vi "wczytajYZ.vi"(7 "Liczba bajtów":u8, 8 "error in (no error)":errorcluster, 9 "I2C Adres":u8, 10 "I2C Kana³":u8, 11 "LINX Resource in":T1) -> (0 "error out":errorcluster, 1 "Oœ Z":dbl[](array[numeric]), 2 "Oœ Y":dbl[](array[numeric]), 3 "LINX Resource out":T1)   [LabVIEW 2014]
uses:
  <vilib>/MakerHub/LINX/Private/Type Defs/LINX Ref.ctl
  <vilib>/MakerHub/LINX/Private/Type Defs/Platform.ctl
  <vilib>/MakerHub/LINX/Private/Type Defs/Interface.ctl
  <vilib>/MakerHub/LINX/Private/Device/Type Defs/LINX Device Config.ctl
  <vilib>/MakerHub/LINX/Private/Device/Type Defs/TCP Config.ctl
  <vilib>/MakerHub/LINX/Private/Device/Type Defs/Channels.ctl
  <vilib>/MakerHub/LINX/Private/Type Defs/Peripherals/I2C/EOF.ctl
  <vilib>/MakerHub/LINX/Private/Local IO/LinxI2cWrite.vi
  <vilib>/MakerHub/LINX/Public/Utilities/Check Channel.vi
  <vilib>/MakerHub/LINX/Private/Local IO/Handle Errors.vi
  <vilib>/MakerHub/LINX/Private/Utilties/Generate Error.vi
  <vilib>/MakerHub/LINX/LMH-LINX.lvlib
  <vilib>/MakerHub/LINX/Private/Device/Device.lvlib
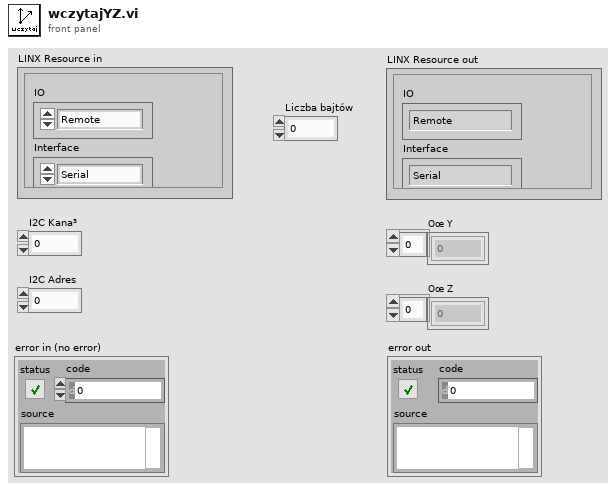
[diagram p1: front panel]
types:
  T1 = typedef "LMH-LINX.lvlib/LINX Ref.ctl" = cluster{"IO":T2, "Interface":T3, "LINX Device Config":T4}
  T2 = typedef "LMH-LINX.lvlib/Platform.ctl" = enum16{"Remote", "Local"}
  T3 = typedef "LMH-LINX.lvlib/Interface.ctl" = enum16{"Serial", "TCP"}
  T4 = typedef "LMH-LINX.lvlib/Device.lvlib/LINX Device Config.ctl" = cluster{"Interface":T3, "COM Port":refnum<visa-resource-name>, "TCP Configuration":T5, "Device Family":u8, "Device ID":u8, "Device Name":string, "TCP Ref":refnum<k5>, "Channels":T6}
  T5 = typedef "LMH-LINX.lvlib/Device.lvlib/TCP Config.ctl" = cluster{"IP Address":string, "Port":u16}
  T6 = typedef "LMH-LINX.lvlib/Channels.ctl" = cluster{"DI":u8[], "DO":u8[], "AI":u8[], "AO":u8[], "PWM":u8[], "QE":u8[], "UART":u8[], "I2C 2":u8[], "SPI":u8[], "CAN":u8[], "Servo":u8[], "AI Ref (V)":dbl, "AI Resolution (Bits)":u8, "AO Ref (V)":dbl, "AO Resolution (Bits)":u8}
  T7 = typedef "LMH-LINX.lvlib/EOF.ctl" = enum8{"Stop", "Restart", "Restart No Stop", "No Stop"}
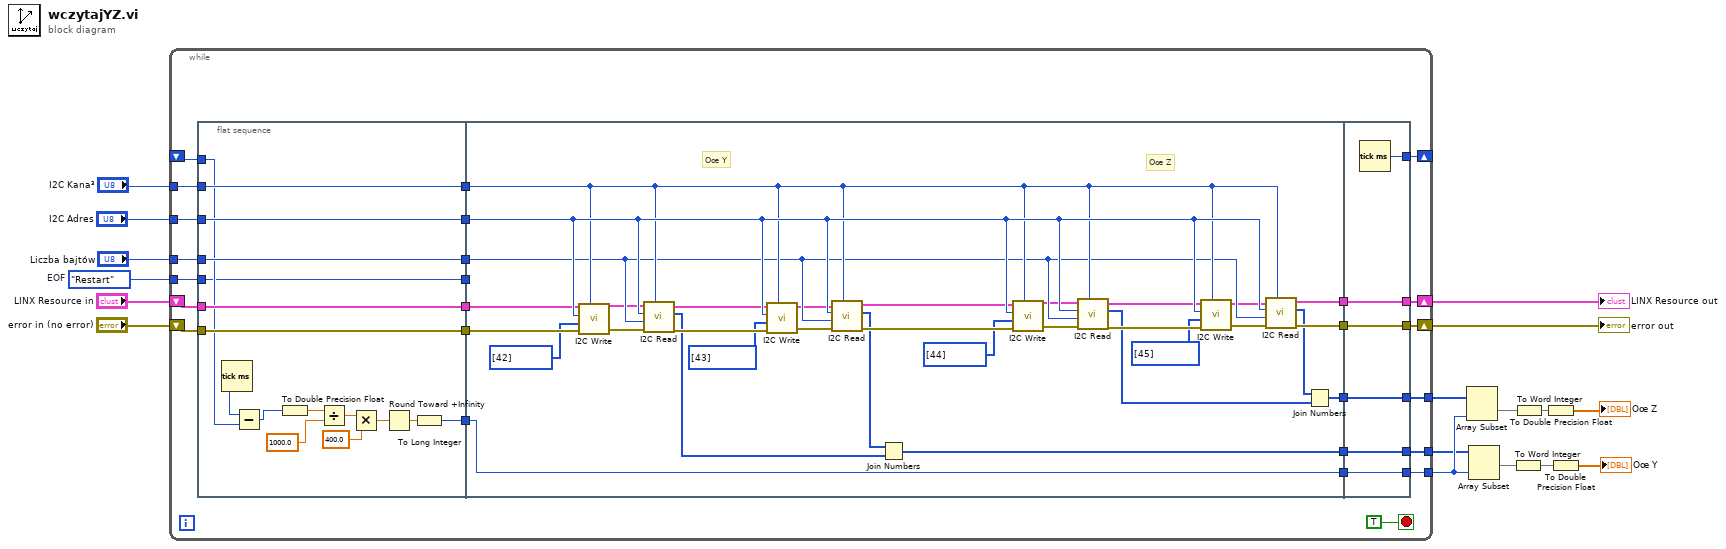
[diagram p0: block diagram]
diagram:
  w1 = EOF."Restart"  # EOF
  n1 = while {
    tunnel: "I2C Adres" -> [w43]
    tunnel: "I2C Kana³" -> [w42]
    tunnel: "Liczba bajtów" -> [w41]
    tunnel: [w38] -> w2
    tunnel: [w35] -> w10
    shift-right: [w36] -> w9
    shift-left: "LINX Resource in" -> [w40]
    shift-right: [w37] -> w8
    shift-left: "error in (no error)" -> [w39]
    shift-right: [w30] -> _
    shift-left: _ -> [w23]
    tunnel: [w20] -> w17
    tunnel: w1 -> [w18]
    stop <- TRUE stop-if-true
    n2 = flat-sequence {
      tunnel: w39 -> [w55]
      tunnel: w40 -> [w56]
      tunnel: w41 -> [w57]
      tunnel: w42 -> [w58]
      tunnel: w43 -> [w59]
      tunnel: [w59] -> w28
      tunnel: [w58] -> w27
      tunnel: [w57] -> w26
      tunnel: [w56] -> w25
      tunnel: [w55] -> w24
      tunnel: w23 -> [w50]
      tunnel: [w49] -> w22
      tunnel: [w44] -> w19
      tunnel: w18 -> [w44]
      tunnel: [w86] -> w34
      tunnel: [w85] -> w33
      tunnel: [w84] -> w32
      tunnel: [w60] -> w31
      tunnel: w28 -> [w91]
      tunnel: w27 -> [w90]
      tunnel: w26 -> [w89]
      tunnel: w25 -> [w88]
      tunnel: w24 -> [w87]
      tunnel: w22 -> [w63]
      tunnel: [w63] -> w21
      tunnel: w19 -> [_]
      tunnel: [w94] -> w35
      tunnel: [w95] -> w36
      tunnel: [w96] -> w37
      tunnel: [w97] -> w38
      tunnel: w34 -> [w97]
      tunnel: w33 -> [w96]
      tunnel: w32 -> [w95]
      tunnel: w31 -> [w94]
      tunnel: [w93] -> w30
      tunnel: [w92] -> w20
      tunnel: w21 -> [w92]
      frame #0 {
        n3 = Tick Count (ms)() -> (millisecond timer value=w51:u32)
        n4 = Subtract(x=w51, y=w50) -> (x-y=w47:u32)
        n5 = To Double Precision Float(number=w47) -> (double precision float=w46:dbl)
        n6 = Divide(x=w46, y=1000.0 ("x")) -> (x/y=w48:dbl)
        n7 = Multiply(x=w48, y=400.0) -> (x*y=w53:dbl)
        n8 = Round Toward +Infinity(x=w53) -> (ceil(x): smallest int >= x=w54:dbl)
        n9 = To Long Integer(number=w54) -> (32bit integer=w49:i32)
      }
      frame #1 {
        # "Oœ Z"
        # "Oœ Y"
        n10 = call <vilib>:"I2C Write.vi"("I2C Channel"=w90, "Error In"=w87, "Data"=u8[] [42], "I2C Slave Address (0)"=w91, "LINX Resource"=w88) -> ("Error Out"=w81:errorcluster, "LINX Resource"=w82:T1)  [unwired: 5 in]
        n11 = call <vilib>:"I2C Read.vi"("I2C Channel"=w90, "Error In"=w81, "Bytes To Read"=w89, "I2C Slave Address (0)"=w91, "LINX Resource"=w82) -> ("Error Out"=w78:errorcluster, "Data"=w62:u8[], "LINX Resource"=w79:T1)  [unwired: 4 in]
        n12 = call <vilib>:"I2C Write.vi"("I2C Channel"=w90, "Error In"=w78, "Data"=u8[] [43], "I2C Slave Address (0)"=w91, "LINX Resource"=w79) -> ("Error Out"=w80:errorcluster, "LINX Resource"=w77:T1)  [unwired: 5 in]
        n13 = call <vilib>:"I2C Read.vi"("I2C Channel"=w90, "Error In"=w80, "Bytes To Read"=w89, "I2C Slave Address (0)"=w91, "LINX Resource"=w77) -> ("Error Out"=w69:errorcluster, "Data"=w61:u8[], "LINX Resource"=w70:T1)  [unwired: 4 in]
        n14 = Join Numbers(hi=w61, lo=w62) -> ((hi.lo)=w60:u16[])
        n15 = call <vilib>:"I2C Write.vi"("I2C Channel"=w90, "Error In"=w69, "Data"=u8[] [44], "I2C Slave Address (0)"=w91, "LINX Resource"=w70) -> ("Error Out"=w75:errorcluster, "LINX Resource"=w76:T1)  [unwired: 5 in]
        n16 = call <vilib>:"I2C Read.vi"("I2C Channel"=w90, "Error In"=w75, "Bytes To Read"=w89, "I2C Slave Address (0)"=w91, "LINX Resource"=w76) -> ("Error Out"=w72:errorcluster, "Data"=w67:u8[], "LINX Resource"=w73:T1)  [unwired: 4 in]
        n17 = call <vilib>:"I2C Write.vi"("I2C Channel"=w90, "Error In"=w72, "Data"=u8[] [45], "I2C Slave Address (0)"=w91, "LINX Resource"=w73) -> ("Error Out"=w74:errorcluster, "LINX Resource"=w71:T1)  [unwired: 5 in]
        n18 = call <vilib>:"I2C Read.vi"("I2C Channel"=w90, "Error In"=w74, "Bytes To Read"=w89, "I2C Slave Address (0)"=w91, "LINX Resource"=w71) -> ("Error Out"=w85:errorcluster, "Data"=w68:u8[], "LINX Resource"=w84:T1)  [unwired: 4 in]
        n19 = Join Numbers(hi=w68, lo=w67) -> ((hi.lo)=w86:u16[])
      }
      frame #2 {
        n20 = Tick Count (ms)() -> (millisecond timer value=w93:u32)
      }
    }
  }
  "LINX Resource out" <- w9
  "error out" <- w8
  n21 = Array Subset(array=w2, length=w17) -> (w15:u16[])  [unwired: 1 in]
  n22 = Array Subset(array=w10, length=w17) -> (w11:u16[])  [unwired: 1 in]
  n23 = To Word Integer(number=w11) -> (16bit integer=w12:i16[])
  n24 = To Word Integer(number=w15) -> (16bit integer=w14:i16[])
  n25 = To Double Precision Float(number=w14) -> (double precision float=→"Oœ Z":dbl[])
  n26 = To Double Precision Float(number=w12) -> (double precision float=→"Oœ Y":dbl[])
